vi "Set gRPC ID.vi"(10 "gRPC ID":T1, 11 "OOP Server in":refnum<class "OCV.lvclass">) -> (3 "OOP Server out":refnum<class "OCV.lvclass">)   [LabVIEW 2019, in "OCV.lvlib" / "OCV.lvclass"]
uses:
  OCV.lvclass
  gRPC lvSupport/Server API/typeDefs/grpcId.ctl
  OCV.lvclass/OCV.ctl
  gRPC lvSupport/gprc-lvsupport.lvlib
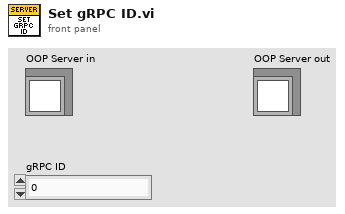
[diagram p1: front panel]
types:
  T1 = typedef "OCV.lvlib/gprc-lvsupport.lvlib/grpcId.ctl" = u64
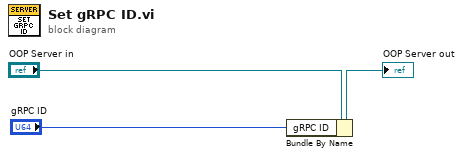
[diagram p0: block diagram]
diagram:
  n1 = Bundle By Name(cluster="OOP Server in", "gRPC ID"="gRPC ID") -> (→"OOP Server out":refnum<class "OCV.lvclass">)
